vi "InitGenericShutdown.vi"() -> (1 "Shutdown Queue":refnum<queue>, 2 "error out":errorcluster)   [LabVIEW 2009]
doc: "Initializes the Generic Shutdown Queue."
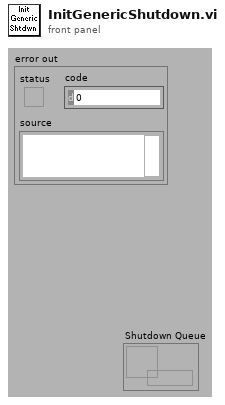
[diagram p1: front panel]
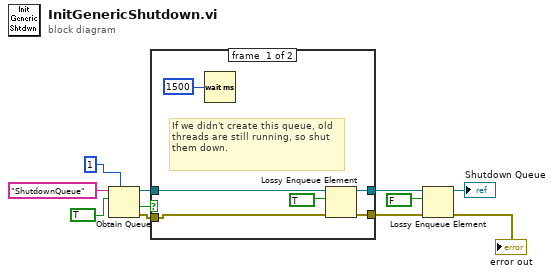
[diagram p0: block diagram]
diagram:
  n1 = Obtain Queue(max queue size (-1, unlimited)=1, name (unnamed)="ShutdownQueue", element data type=TRUE ("create if not found? (T)")) -> (queue out=w7:refnum<queue>, created new?=w8:bool, error out=w3:errorcluster)  [unwired: 2 in]
  n2 = case shown="True" w8 {
    tunnel: w7 -> [w17 w19]
    tunnel: [w14 w19] -> w4
    tunnel: w3 -> [w13 w18]
    tunnel: [w12 w18] -> w2
    frame #0 {
      # "If we didn't create this queue, old threads are still running, so shut them down."
      n3 = Wait (ms)(milliseconds to wait=u32 1500) -> ()  [unwired: 1 out]
      n4 = Lossy Enqueue Element(queue=w17, element=TRUE, error in (no error)=w13) -> (queue out=w14:refnum<queue>, error out=w12:errorcluster)  [unwired: 2 out]
    }
    frame #1 {
    }
  }
  n5 = Lossy Enqueue Element(queue=w4, element=FALSE, error in (no error)=w2) -> (queue out=→"Shutdown Queue":refnum<queue>, error out=→"error out":errorcluster)  [unwired: 2 out]
